vi "BlinkM ReadScriptLine.vi"(7 "Script Line (0)":u8, 8 "Error In":errorcluster, 9 "BlinkM Script (User Script)":T5, 10 "Address (0)":u8, 11 "Arduino Resource":T1={"COM Port"="", "Board Type"=enum."ChipKit uC32", "Connection Type"=enum."USB / Serial", "Baud Rate (115200)"=15, "Bytes Per Packet (15)"=15, "DI Port Num Pins"=0, "DO Port Num Pins"=0}) -> (0 "Error Out":errorcluster, 2 "BlinkM Script Line":T4, 3 "Arduino Resource":T1={"COM Port"="", "Board Type"=enum."ChipKit uC32", "Connection Type"=enum."USB / Serial", "Baud Rate (115200)"=15, "Bytes Per Packet (15)"=15, "DI Port Num Pins"=0, "DO Port Num Pins"=0})   [LabVIEW 2011, in "LabVIEW Interface for ChipKit.lvlib"]
doc: "Read a light script line from the specified BlinkM."
uses:
  LabVIEW Interface for ChipKit.lvlib
  Private/Type Defs/BlinkM Script.ctl
  Private/Type Defs/BlinkM Script Line.ctl
  Private/Type Defs/Chipkit Resource.ctl
  Private/Type Defs/Board Type.ctl
  Private/Type Defs/Connection Type.ctl
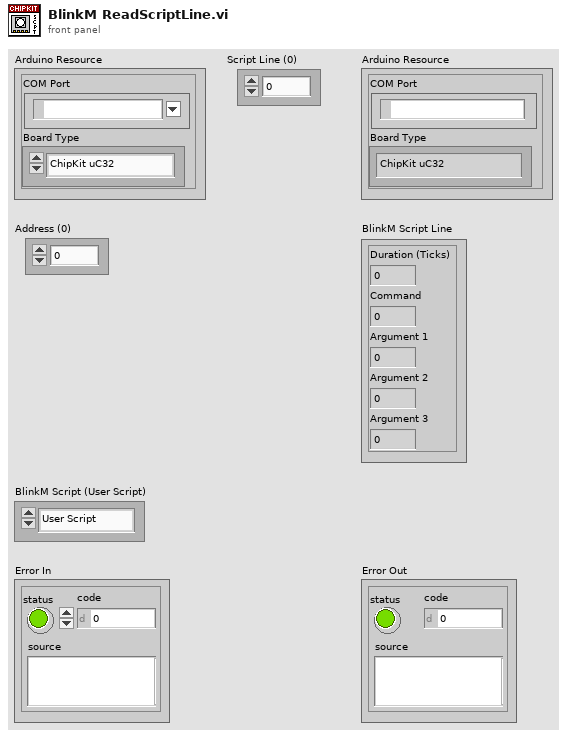
[diagram p1: front panel]
types:
  T1 = typedef "LabVIEW Interface for ChipKit.lvlib/Chipkit Resource.ctl" = cluster{"COM Port":refnum<visa-resource-name>, "Board Type":T2, "Connection Type":T3, "Baud Rate (115200)":u32, "Bytes Per Packet (15)":u32, "DI Port Num Pins":i32, "DO Port Num Pins":i32}
  T2 = typedef "LabVIEW Interface for ChipKit.lvlib/Board Type.ctl" = enum16{"ChipKit uC32", "ChipKit Uno32", "ChipKit Max32"}
  T3 = typedef "LabVIEW Interface for ChipKit.lvlib/Connection Type.ctl" = enum8{"USB / Serial", "XBEE", "BlueSmirf (Bluetooth)"}
  T4 = typedef "LabVIEW Interface for ChipKit.lvlib/BlinkM Script Line.ctl" = cluster{"Duration (Ticks)":u8, "Command":u8, "Argument 1":u8, "Argument 2":u8, "Argument 3":u8}
  T5 = typedef "LabVIEW Interface for ChipKit.lvlib/BlinkM Script.ctl" = enum8{"User Script", "RGB", "White Flash", "Red Flash", "Green Flash", "Blue Flash", "Cyan Flash", "Magenta Flash", "Yellow Flash", "Black", "Hue Cycle", "Mood Light", "Virtual Candle", "Water Reflections", "Old Neon", "The Seasons", "Thunderstorm", "Stop Light", "Morse Code S.O.S"}
  T6 = cluster{"Duration (Ticks)":u8, "Command":u8, "Argument 1":u8, "Argument 2":u8, "Argument 3":u8}
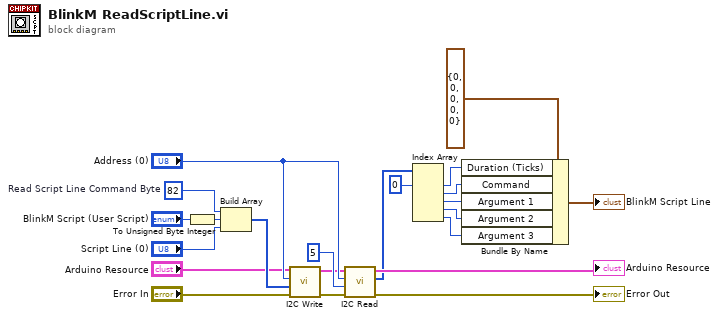
[diagram p0: block diagram]
diagram:
  w21 = u8 82  # Read Script Line Command Byte
  n1 = To Unsigned Byte Integer(number="BlinkM Script (User Script)") -> (unsigned 8bit integer=w7:u8)
  n2 = Build Array(w21, w7, "Script Line (0)") -> (w20:u8[])
  n3 = call "I2C Write.vi"("Error In"="Error In", "I2C Data"=w20, "Address (0)"="Address (0)", "ChipKit Resource"="Arduino Resource") -> ("Error Out"=w18:errorcluster, "ChipKit Resource"=w3:T1)  [unwired: 6 in]
  n4 = call "I2C Read.vi"("Error In"=w18, "Bytes To Read"=u8 5, "Address (0)"="Address (0)", "ChipKit Resource"=w3) -> ("Error Out"=→"Error Out":errorcluster, "I2C Data"=w1:u8[], "ChipKit Resource"=→"Arduino Resource":T1)  [unwired: 5 in]
  n5 = Index Array(array=w1, index #1=0 ("index")) -> (element #1=w13:u8, element #2=w12:u8, element #3=w11:u8, element #4=w10:u8, element #5=w9:u8)  [unwired: 4 in]
  n6 = Bundle By Name(cluster=T6 {"Duration (Ticks)"=0, "Command"=0, "Argument 1"=0, "Argument 2"=0, "Argument 3"=0}, "Duration (Ticks)"=w13, "Command"=w12, "Argument 1"=w11, "Argument 2"=w10, "Argument 3"=w9) -> (→"BlinkM Script Line":T6)
